vi "Decode Topic Subscriptions.vi"(10 "Payload":u8[](array[numeric]) format="%08b") -> (1 "Valid?":bool, 2 "Topic Subscriptions":string[](array[string]))   [LabVIEW 2013, in "UNSUBSCRIBE.lvclass"]
uses:
  UNSUBSCRIBE.lvclass
  ControlPacket/ControlPacket.lvclass
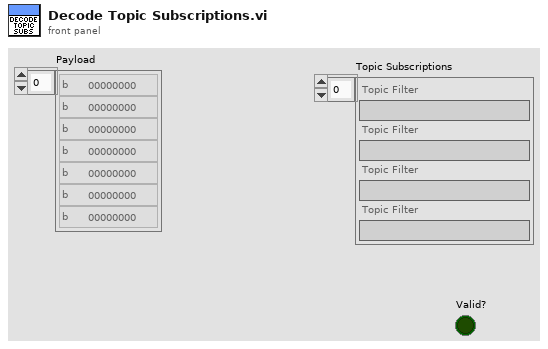
[diagram p1: front panel]
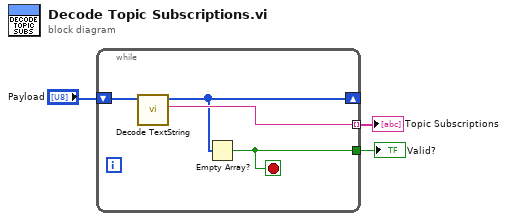
[diagram p0: block diagram]
diagram:
  n1 = while {
    shift-right: [w5] -> _
    shift-left: "Payload" -> [w7]
    tunnel: [w6] -> w1 mode=indexing
    tunnel: [w4] -> w3
    stop <- w4 stop-if-true
    n2 = call "Decode TextString.vi"("Length-Prefixed Field"=w7) -> ("Text String"=w6:string, "Remaining Packets"=w5:u8[])  [unwired: 9 in]
    n3 = Empty Array?(array=w5) -> (empty?=w4:bool)
  }
  "Valid?" <- w3
  "Topic Subscriptions" <- w1
